vi "Write Clients.vi"(8 "error in":errorcluster, 10 "Clients":T1[](array[typedef]), 11 "System in":refnum<class "System.lvclass">) -> (0 "error out":errorcluster, 3 "System out":refnum<class "System.lvclass">)   [LabVIEW 2014, in "System.lvclass"]
uses:
  System.lvclass
  Controls/Client Ref.ctl
  System.lvclass/System.ctl
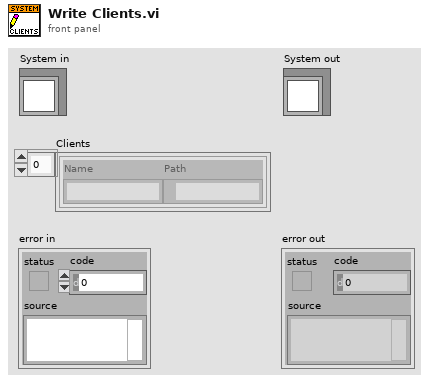
[diagram p1: front panel]
types:
  T1 = typedef "Client Ref.ctl" = cluster{"Name":string, "Path":path}
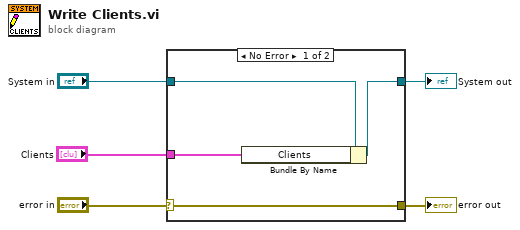
[diagram p0: block diagram]
diagram:
  n1 = case shown="No Error" "error in" {
    selector: "error in" -> [w9 w10]
    tunnel: [w9 w10] -> w4
    tunnel: [w7 w11] -> w2
    tunnel: "System in" -> [w8 w11]
    tunnel: "Clients" -> [w6 _]
    frame No Error {
      n2 = Bundle By Name(cluster=w8, "Clients"=w6) -> (w7:refnum<class "System.lvclass">)
    }
    frame Error {
    }
  }
  "error out" <- w4
  "System out" <- w2
